vi "Vision Save.vi"(11 "Save":refnum<vi>) -> ()   [LabVIEW 2023]
uses:
  <vilib>/Rock Robotics/Network Tables/NT Read Boolean.vi
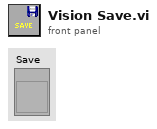
[diagram p1: front panel]
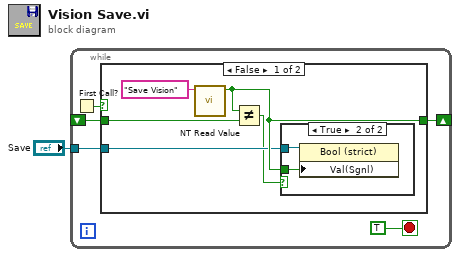
[diagram p0: block diagram]
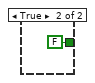
[diagram p3: hidden frame]
diagram:
  n1 = while {
    shift-right: [w5] -> _
    shift-left: _ -> [w4]
    tunnel: "Save" -> [w3]
    stop <- TRUE stop-if-true
    n2 = First Call?() -> (First Call?: T/F=w6:bool)
    n3 = case shown="False" w6 {
      tunnel: [w9 FALSE ("Boolean")] -> w5
      tunnel: w4 -> [w10 _]
      tunnel: w3 -> [w8 _]
      frame False {
        n4 = call-poly <vilib>:"NT Read Value.vi"("name"="Save Vision" ("Name")) -> ("value"=w9:bool)  [unwired: 8 in, 2 out]
        n5 = Not Equal?(x=w9, y=w10) -> (x != y?=w7:bool)
        n6 = case shown="True" w7 {
          tunnel: w9 -> [_ w13]
          tunnel: w8 -> [_ w12]
          frame False {
          }
          frame True {
            n7 = property on="Property Node" class="Bool (strict)"(reference=w12, "Val(Sgnl)"=w13) -> ()  [unwired: 1 in, 2 out]
          }
        }
      }
      frame True {
      }
    }
  }
